vi "gentec-M-Link.Stop Data Flow.vi"(0 "VISA resource In":refnum<visa-resource-name>, 5 "error in (no error)":errorcluster) -> (11 "Data Read":string, 13 "Read Timeout":bool, 14 "VISA resource Out":refnum<visa-resource-name>, 16 "Success":bool, 19 "error out":errorcluster)   [LabVIEW 2014, in "gentec-M-Link - Driver.lvlib"]
doc: "Data to write: str0\n\nStops the data flow and replies ok."
uses:
  gentec-M-Link - Driver.lvlib
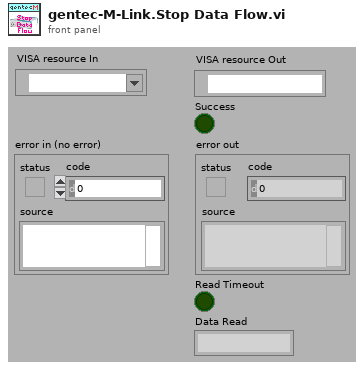
[diagram p1: front panel]
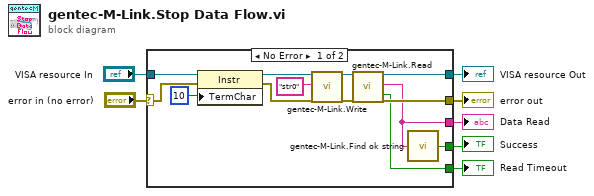
[diagram p0: block diagram]
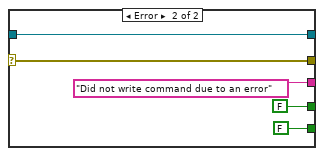
[diagram p2: hidden frame]
diagram:
  n1 = case shown="No Error" "error in (no error)" {
    selector: "error in (no error)" -> [w14 w25]
    tunnel: [w18 w25] -> w6
    tunnel: "VISA resource In" -> [w16 w24]
    tunnel: [w20 w24] -> w4
    tunnel: [w19 FALSE ("Found")] -> w3
    tunnel: [w9 "Did not write command due to an error" ("Data Read")] -> w2
    tunnel: [w8 FALSE ("Read Timeout")] -> w1
    frame No Error {
      n2 = property class="Instr"(reference=w16, error in=w14, "TermChar"=u8 10 ("Message Based Settings:Termination Character")) -> (reference out=w15:refnum<visa-resource-name>, error out=w13:errorcluster)
      n3 = call "gentec-M-Link.Write.vi"("VISA resource (In)"=w15, "Data To Write"="str0", "error in (no error)"=w13) -> ("VISA resource (Out)"=w11:refnum<visa-resource-name>, "error out"=w10:errorcluster)  [unwired: 14 in, 1 out]
      n4 = call "gentec-M-Link.Read.vi"("VISA resource (In)"=w11, "error in (no error)"=w10) -> ("VISA resource (Out)"=w20:refnum<visa-resource-name>, "Data Read"=w9:string, "Read Timeout"=w8:bool, "error out"=w18:errorcluster)  [unwired: 13 in, 1 out]
      n5 = call "gentec-M-Link.Find ok string.vi"("string"=w9) -> ("Found"=w19:bool)
    }
    frame Error {
    }
  }
  "error out" <- w6
  "VISA resource Out" <- w4
  "Success" <- w3
  "Data Read" <- w2
  "Read Timeout" <- w1
